vi "Leaktest Read Config 05.vi"(6 "error in (no error)":errorcluster, 8 "Cfg Filename":string="Leaktest.ini", 9 "File Location":T5={"Cfg directory type"=3, "Rel Log Path"="LeakTest"} {"Cfg directory type" items=["User Home"=0, "User Desktop"=1, "User Documents"=2, "User Application Data"=3, "User Preferences"=4, "User Temporary"=5, "Public Documents"=6, "Public Application Data"=7, "Public Preferences"=8, "Public Cache"=13, "System Core Libraries"=9, "System Installed Libraries"=10, "Application Files"=11, "Boot Volume Root"=12]}) -> (0 "error out":errorcluster, 2 "Config Clst":T1={"Log Dir Path"=path "\\\\spa-mu2e-network\\Files/LeakRateRawData", "File Log Sec"=30.0, "34970A Sec"=1.0, "Chart hrs1"=0.25, "Chart hrs2"=0.25, "Filnen Fmt"="%y%m%d_%H%M_MN#.txt", "Temp chans"="Dev1/Ti0, Dev1/Ti2, Dev1/Ti4", "DI Lines"="Dev1/AuxPort/Di2:3", "DO Lines"="Dev1/AuxPort/Do0:1", "VISA ID 34970A"="34970A", "Baud Rate"=enum."38400", "Time Fmt"=enum."Days"} {"Chart hrs2" format="%.1f"; "Chart hrs1" format="%.1f"; "34970A Sec" format="%.1f"; "File Log Sec" format="%.1f"}, 3 "Config Filepath":path, 4 "Press Scaling":T2(array[cluster])=[{"Gain"=7.5, "Offset"=-7.5, "Units"="PSI", "Channel"="101", "Name"="Fill 1"}, {"Gain"=7.5, "Offset"=-7.5, "Units"="PSI", "Channel"="102", "Name"="Ref 1"}, {"Gain"=2.0, "Offset"=0.0, "Units"="H2O", "Channel"="103", "Name"="Diff 1"}, {"Gain"=7.5, "Offset"=7.5, "Units"="PSI", "Channel"="104", "Name"="Fill 2"}, {"Gain"=7.5, "Offset"=-7.46, "Units"="PSI", "Channel"="105", "Name"="Ref 2"}, {"Gain"=2.0, "Offset"=-0.038, "Units"="H2O", "Channel"="106", "Name"="Diff 2"}], 5 "Control Params":T3={"Setpt C"=24.0, "PID"={" gain (Kc)"=180.0, "integral min"=5.0, "derivative min"=0.0}} {"Setpt C" format="%.2f"; "PID"."derivative min" format="%.3f"; "PID"."integral min" format="%.3f"; "PID"."gain (Kc)" format="%.3f"})   [LabVIEW 2020]
uses:
  System Directory Type.ctl
  Cfg Cluster Typedef.ctl
panel:
  # "Don't change name or channel"
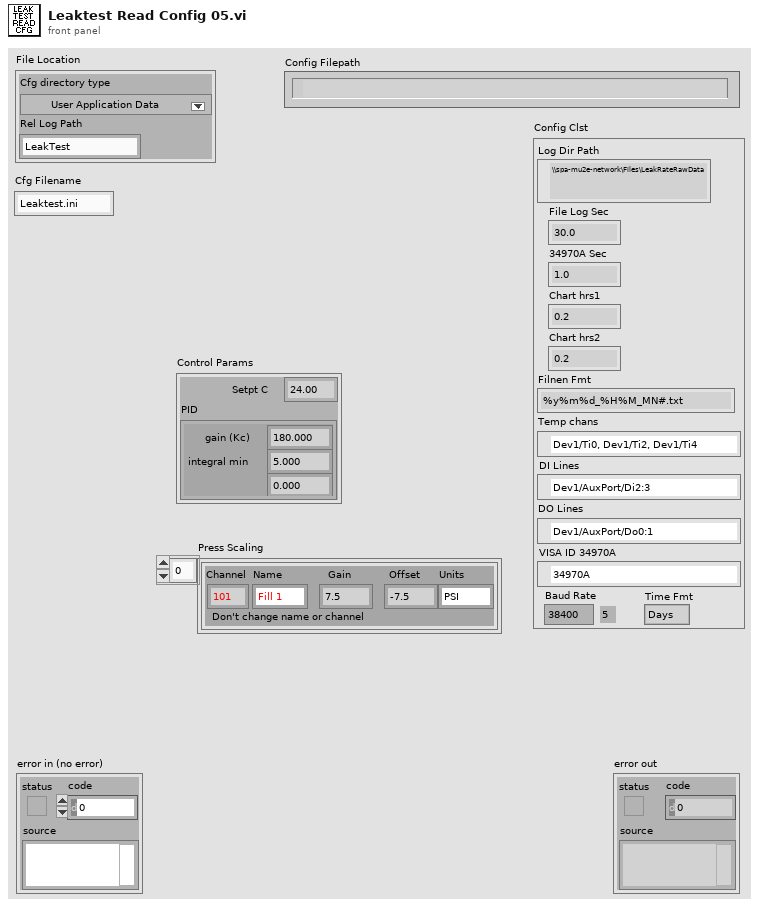
[diagram p1: front panel]
types:
  T1 = typedef "Cfg Cluster Typedef.ctl" = cluster{"Log Dir Path":path, "File Log Sec":dbl, "34970A Sec":dbl, "Chart hrs1":dbl, "Chart hrs2":dbl, "Filnen Fmt":string, "Temp chans":refnum<k21>, "DI Lines":refnum<k21>, "DO Lines":refnum<k21>, "VISA ID 34970A":refnum<visa-resource-name>, "Baud Rate":enum16{"1200", "2400", "4800", "9600", "19200", "38400", "57600", "115200"}, "Time Fmt":enum16{"H:M:S", "Days", "Secs"}}
  T2 = cluster{"Gain":dbl, "Offset":dbl, "Units":string, "Channel":string, "Name":string}[]
  T3 = cluster{"Setpt C":dbl, "PID":cluster{" gain (Kc)":dbl, "integral min":dbl, "derivative min":dbl}}
  T4 = typedef "System Directory Type.ctl" = i32
  T5 = cluster{"Cfg directory type":T4, "Rel Log Path":string}
  T6 = cluster{"[0]":string, "[1]":string, "[2]":string, "[3]":string, "[4]":string}
  T7 = cluster{"[0]":string, "[1]":string, "[2]":string}
  T8 = cluster{"[0]":dbl, "[1]":dbl, "[2]":dbl, "[3]":dbl}
  T9 = cluster{"Gain":dbl, "Offset":dbl, "Units":string, "Channel":string, "Name":string}
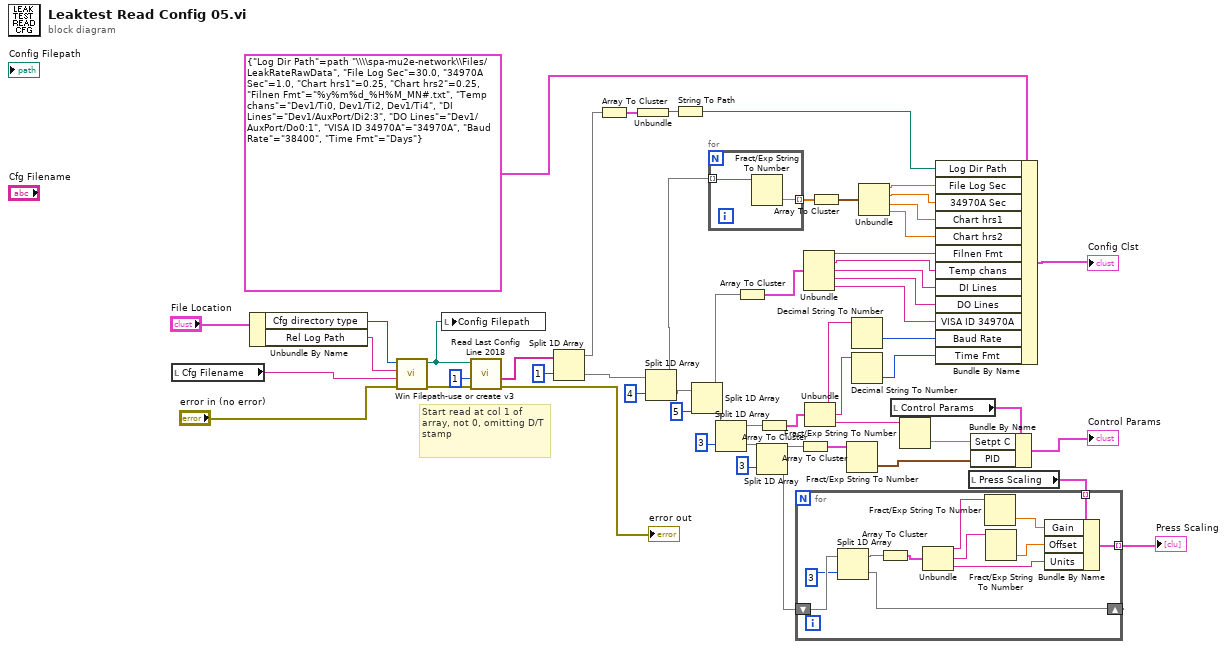
[diagram p0: block diagram]
diagram:
  # "Start read at col 1 of array, not 0, omitting D/T stamp"
  n1 = local read "Cfg Filename"() -> (w17:string)
  n2 = Unbundle By Name("File Location") -> ("Cfg directory type"=w19:T4, "Rel Log Path"=w18:string)
  n3 = call "Win Filepath-use or create v3.vi"("error in"="error in (no error)", "File Name"=w17, "Subdir"=w18, "Win Directory Type"=w19) -> ("error out"=w21:errorcluster, "Filepath"=w15:path)  [unwired: 4 in]
  n4 = local write "Config Filepath"(w15) -> ()
  n5 = call "Read Last Config Line 2018.vi"("error in (no error)"=w21, "Start Col"=1, "Test Config path"=w15) -> ("error out"=→"error out":errorcluster, "1d Out"=w23:string[])  [unwired: 3 in, 2 out]
  n6 = Split 1D Array(array=w23, index=1) -> (first subarray=w22:string[], second subarray=w25:string[])
  n7 = Array To Cluster(array=w22) -> (cluster=w13:cluster{"[0]":string})
  n8 = Unbundle(w13) -> ("[0]"=w12:string)
  n9 = Split 1D Array(array=w25, index=4) -> (first subarray=w53:string[], second subarray=w48:string[])
  n10 = String To Path(string=w12) -> (path=w11:path)
  n11 = Split 1D Array(array=w48, index=5) -> (first subarray=w45:string[], second subarray=w43:string[])
  n12 = for {
    tunnel: w53 -> [w57] mode=indexing
    tunnel: [w56] -> w52 mode=indexing
    n13 = Fract/Exp String To Number(string=w57) -> (number=w56:dbl)  [unwired: 3 in, 1 out]
  }
  n14 = Split 1D Array(array=w43, index=3) -> (first subarray=w42:string[], second subarray=w36:string[])
  n15 = Array To Cluster(array=w45) -> (cluster=w46:T6)
  n16 = Split 1D Array(array=w36, index=3) -> (first subarray=w35:string[], second subarray=w31:string[])
  n17 = Array To Cluster(array=w42) -> (cluster=w50:T7)
  n18 = Array To Cluster(array=w35) -> (cluster=w34:T7)
  n19 = Unbundle(w46) -> ("[0]"=w6:string, "[1]"=w5:string, "[2]"=w4:string, "[3]"=w3:string, "[4]"=w2:string)
  n20 = Unbundle(w50) -> ("[0]"=w29:string, "[1]"=w28:string, "[2]"=w27:string)
  n21 = Array To Cluster(array=w52) -> (cluster=w51:T8)
  n22 = Fract/Exp String To Number(string=w34) -> (number=w33:cluster{"[0]":dbl, "[1]":dbl, "[2]":dbl})  [unwired: 3 in, 1 out]
  n23 = Decimal String To Number(string=w29) -> (number=w44:i32)  [unwired: 2 in, 1 out]
  n24 = Decimal String To Number(string=w28) -> (number=w26:i32)  [unwired: 2 in, 1 out]
  n25 = Unbundle(w51) -> ("[0]"=w10:dbl, "[1]"=w9:dbl, "[2]"=w8:dbl, "[3]"=w7:dbl)
  n26 = local read "Control Params"() -> (w40:T3)
  n27 = Fract/Exp String To Number(string=w27) -> (number=w38:dbl)  [unwired: 3 in, 1 out]
  n28 = Bundle By Name(cluster=T1 {"Log Dir Path"=path "\\\\spa-mu2e-network\\Files/LeakRateRawData", "File Log Sec"=30.0, "34970A Sec"=1.0, "Chart hrs1"=0.25, "Chart hrs2"=0.25, "Filnen Fmt"="%y%m%d_%H%M_MN#.txt", "Temp chans"="Dev1/Ti0, Dev1/Ti2, Dev1/Ti4", "DI Lines"="Dev1/AuxPort/Di2:3", "DO Lines"="Dev1/AuxPort/Do0:1", "VISA ID 34970A"="34970A", "Baud Rate"=enum."38400", "Time Fmt"=enum."Days"} ("Config Clst"), "Log Dir Path"=w11, "File Log Sec"=w10, "34970A Sec"=w9, "Chart hrs1"=w8, "Chart hrs2"=w7, "Filnen Fmt"=w6, "Temp chans"=w5, "DI Lines"=w4, "DO Lines"=w3, "VISA ID 34970A"=w2, "Baud Rate"=w44, "Time Fmt"=w26) -> (→"Config Clst":T1)
  n29 = local read "Press Scaling"() -> (w32:T2)
  n30 = for {
    shift-right: [w66] -> _
    shift-left: w31 -> [w69]
    tunnel: w32 -> [w67] mode=indexing
    tunnel: [w65] -> w30 mode=indexing
    n31 = Split 1D Array(array=w69, index=3 ("length")) -> (first subarray=w64:string[], second subarray=w66:string[])
    n32 = Array To Cluster(array=w64) -> (cluster=w63:T7)
    n33 = Unbundle(w63) -> ("[0]"=w62:string, "[1]"=w61:string, "[2]"=w60:string)
    n34 = Fract/Exp String To Number(string=w62) -> (number=w58:dbl)  [unwired: 3 in, 1 out]
    n35 = Fract/Exp String To Number(string=w61) -> (number=w59:dbl)  [unwired: 3 in, 1 out]
    n36 = Bundle By Name(cluster=w67, "Gain"=w58, "Offset"=w59, "Units"=w60) -> (w65:T9)
  }
  "Press Scaling" <- w30
  n37 = Bundle By Name(cluster=w40, "Setpt C"=w38, "PID"=w33) -> (→"Control Params":T3)
